vi "Add to Project.vi"(8 "error in (no error)":errorcluster, 11 "Concrete Message Rescripter in":refnum<class "Concrete Message Rescripter.lvclass">) -> (0 "error out":errorcluster, 3 "Concrete Message Rescripter out":refnum<class "Concrete Message Rescripter.lvclass">)   [LabVIEW 2020, in "Message Rescripter.lvlib" / "Concrete Message Rescripter.lvclass"]
uses:
  Concrete Message Rescripter.lvclass
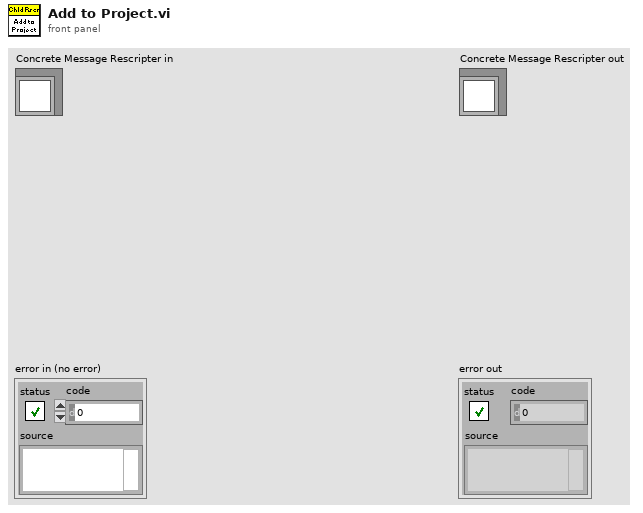
[diagram p1: front panel]
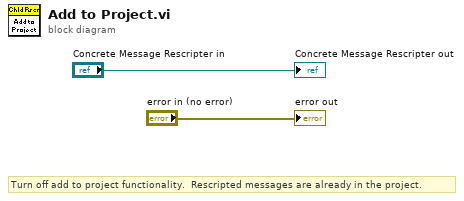
[diagram p0: block diagram]
diagram:
  # "Turn off add to project functionality.  Rescripted messages are already in the project."
  "error out" <- "error in (no error)"
  "Concrete Message Rescripter out" <- "Concrete Message Rescripter in"
